vi "Get Serial Port Config.vi"() -> (0 "error out":errorcluster, 3 "value":string)   [LabVIEW 2020, in "ESP301.lvlib"]
uses:
  ESP301.lvlib
  <vilib>/Utility/config.llb/Read Key (String).vi
  <vilib>/Utility/config.llb/NI_LVConfig.lvlib
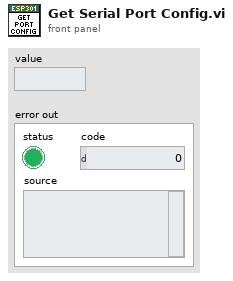
[diagram p1: front panel]
types:
  T1 = typedef "NI_LVConfig.lvlib/Config Data RefNum.ctl" = refnum<k1>
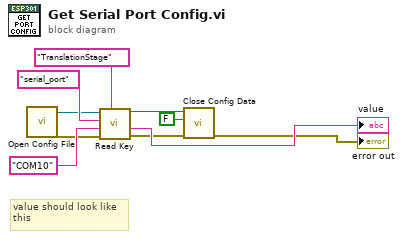
[diagram p0: block diagram]
diagram:
  # "value should look like\nthis"
  n1 = call "Open Config File.vi"() -> ("error out"=w2:errorcluster, "Refnum out"=w1:T1)  [unwired: 10 in]
  n2 = call-poly <vilib>:"Read Key.vi"("section"="TranslationStage", "error in (no error)"=w2, "default value"="COM10", "key"="serial_port", "refnum"=w1) -> ("error out"=w6:errorcluster, "value"=→"value":string, "refnum out"=w7:T1)  [unwired: 3 in, 1 out]
  n3 = call <vilib>:"Close Config Data.vi"("error in (no error)"=w6, "write file if changed (T)"=FALSE, "refnum"=w7) -> ("error out"=→"error out":errorcluster)  [unwired: 7 in, 1 out]
